vi "Generic command handler.vi"(8 "error in (no error)":errorcluster, 10 "Message in":refnum<class "GenericMessage.lvclass">, 11 "TomoConversion in":refnum<class "TomoConversion.lvclass">) -> (0 "error out":errorcluster, 2 "value":string, 3 "TomoConversion out":refnum<class "TomoConversion.lvclass">)   [LabVIEW 2012, in "TomoConversion.lvclass"]
doc: "The generic_command_handler processes the command 'generic'. Commands which are not part of the predefined list of commands fall under the 'generic' command for special activity."
uses:
  TomoConversion.lvclass
  <vilib>/Distrio/Murmex/GenericMessage/GenericMessage.lvclass
  <vilib>/Distrio/Murmex/Murmex/Murmex.lvclass
  TomoConversion.lvclass/TomoConversion.ctl
  <vilib>/Distrio/Murmex/Message/Add or replace parameter.vi
panel:
  # "This method is called when the GENERIC\ntrigger is sent. \n\nOverride this method when your component needs to\nrespond to this trigger. \n\nCall parent for proper implementation"
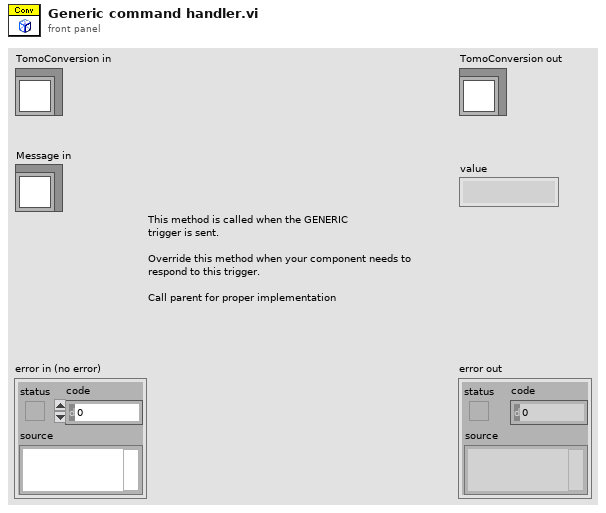
[diagram p1: front panel]
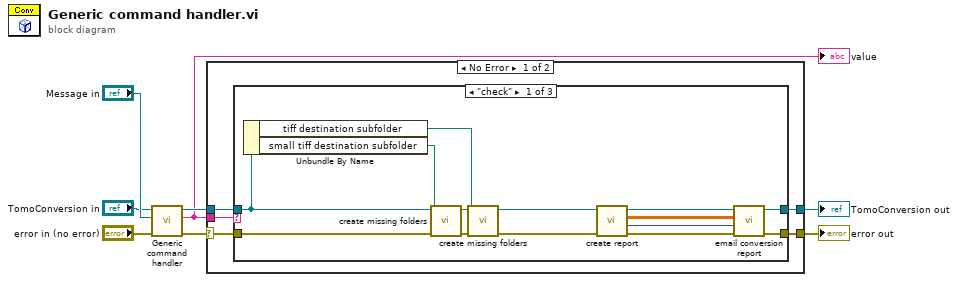
[diagram p0: block diagram]
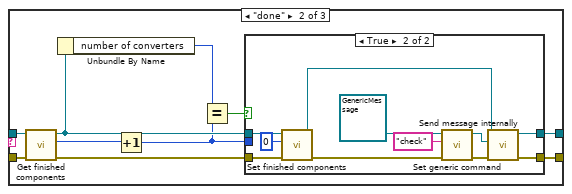
[diagram p2: hidden frame]
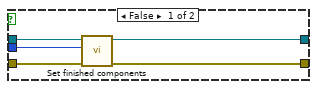
[diagram p3: hidden frame]
diagram:
  n1 = call-parent "Generic command handler.vi"("error in (no error)"="error in (no error)", "Message in"="Message in", "Murmex in"="TomoConversion in") -> ("error out"=w5:errorcluster, "value"=w1:string, "Murmex out"=w4:refnum<class "TomoConversion.lvclass">)  [unwired: 6 in]
  "value" <- w1
  n2 = case shown="No Error" w5 {
    selector: w5 -> [w13 w57]
    tunnel: w4 -> [w10 w56]
    tunnel: w1 -> [w12 _]
    tunnel: [w11 w57] -> w3
    tunnel: [w9 w56] -> w2
    frame No Error {
      n3 = case shown="\"check\"" w12 {
        tunnel: w13 -> [w25 w37 w55]
        tunnel: [w18 w28 w55] -> w11
        tunnel: w10 -> [w26 w36 w54]
        tunnel: [w20 w29 w54] -> w9
        frame "check" {
          n4 = Unbundle By Name(w26) -> ("tiff destination subfolder"=w22:path, "small tiff destination subfolder"=w23:path)
          n5 = call-dynamic "create missing folders.vi"("error in (no error)"=w25, "path"=w23, "TomoConversion in"=w26) -> ("error out"=w24:errorcluster, "TomoConversion out"=w27:refnum<class "TomoConversion.lvclass">)  [unwired: 7 in]
          n6 = call-dynamic "create missing folders.vi"("error in (no error)"=w24, "path"=w22, "TomoConversion in"=w27) -> ("error out"=w14:errorcluster, "TomoConversion out"=w15:refnum<class "TomoConversion.lvclass">)  [unwired: 7 in]
          n7 = call-dynamic "create report.vi"("error in (no error)"=w14, "TomoConversion in"=w15) -> ("error out"=w19:errorcluster, "correct number of subfolders"=w16:i32, "Array"=w17:dbl[][], "TomoConversion out"=w21:refnum<class "TomoConversion.lvclass">)  [unwired: 6 in]
          n8 = call-dynamic "email conversion report.vi"("error in (no error)"=w19, "correct number of subfolders"=w16, "Array"=w17, "TomoConversion in"=w21) -> ("error out"=w18:errorcluster, "TomoConversion out"=w20:refnum<class "TomoConversion.lvclass">)  [unwired: 6 in]
        }
        frame "done" {
          n9 = call-dynamic "Get finished components.vi"("error in (no error)"=w37, "TomoConversion in"=w36) -> ("error out"=w35:errorcluster, "finished components"=w34:u32, "TomoConversion out"=w33:refnum<class "TomoConversion.lvclass">)  [unwired: 7 in]
          n10 = Unbundle By Name(w33) -> ("number of converters"=w32:u32)
          n11 = Increment(x=w34) -> (x+1=w30:u32)
          n12 = Equal?(x=w32, y=w30) -> (x = y?=w31:bool)
          n13 = case shown="True" w31 {
            tunnel: w35 -> [w42 w51]
            tunnel: w33 -> [w41 w53]
            tunnel: w30 -> [w40 _]
            tunnel: [w39 w43] -> w29
            tunnel: [w38 w50] -> w28
            frame False {
              n14 = call-dynamic "Set finished components.vi"("error in (no error)"=w42, "finished components"=w40, "TomoConversion in"=w41) -> ("error out"=w38:errorcluster, "TomoConversion out"=w39:refnum<class "TomoConversion.lvclass">)  [unwired: 7 in]
            }
            frame True {
              n15 = call-dynamic "Set finished components.vi"("error in (no error)"=w51, "finished components"=u32 0, "TomoConversion in"=w53) -> ("error out"=w46:errorcluster, "TomoConversion out"=w48:refnum<class "TomoConversion.lvclass">)  [unwired: 7 in]
              n16 = call <vilib>:"Set generic command.vi"("error in (no error)"=w46, "generic command"="check", "GenericMessage in"=refnum<class "GenericMessage.lvclass"> refnum ("Message in")) -> ("error out"=w47:errorcluster, "GenericMessage out"=w49:refnum<class "GenericMessage.lvclass">)  [unwired: 7 in]
              n17 = call <vilib>:"Send message internally.vi"("error in (no error)"=w47, "Message"=w49, "Murmex in"=w48) -> ("error out"=w50:errorcluster, "Murmex out"=w43:refnum<class "TomoConversion.lvclass">)  [unwired: 7 in]
            }
          }
        }
        frame Default {
        }
      }
    }
    frame Error {
    }
  }
  "error out" <- w3
  "TomoConversion out" <- w2
